vi "XYZStage-Z-axis safety interlock.vi"(7 "Interlock check type":T1, 8 "error in (no error)":errorcluster, 10 "Z move to":sgl, 11 "Z Current":sgl) -> (0 "error out":errorcluster, 3 "Z":sgl)   [LabVIEW 2020]
uses:
  Typedefs/Z intelock check type.ctl
  User Interface/Windows/Position control window/Globals/Pos ctrl window globals.vi
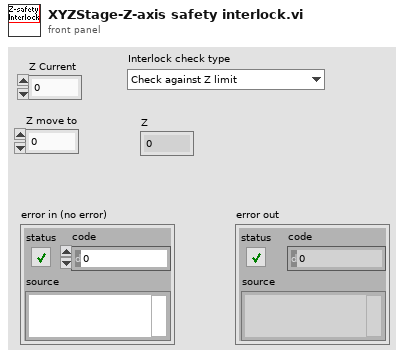
[diagram p1: front panel]
types:
  T1 = typedef "Z intelock check type.ctl" = enum16{"Check against Z limit", "Check againt current position"}
  T2 = typedef "Imaging Protocols enum.ctl" = enum16{"AOL Z-Stack", "Motor Z Stack", "Parameter Sweep", "Functional Acquisition", "Single Plane Acquisition", "Volume Acquisition", "Live Imaging", "Live Plane Imaging", "Live Volume Imaging"}
  T3 = cluster{"Caption-Right button":string, "Caption-Left button":string, "Message to display":string, "Delay before close":u32, "Window Colour":u32, "Cancel button disabled?":enum8{"Enabled", "Disabled", "Disabled and Grayed Out"}}
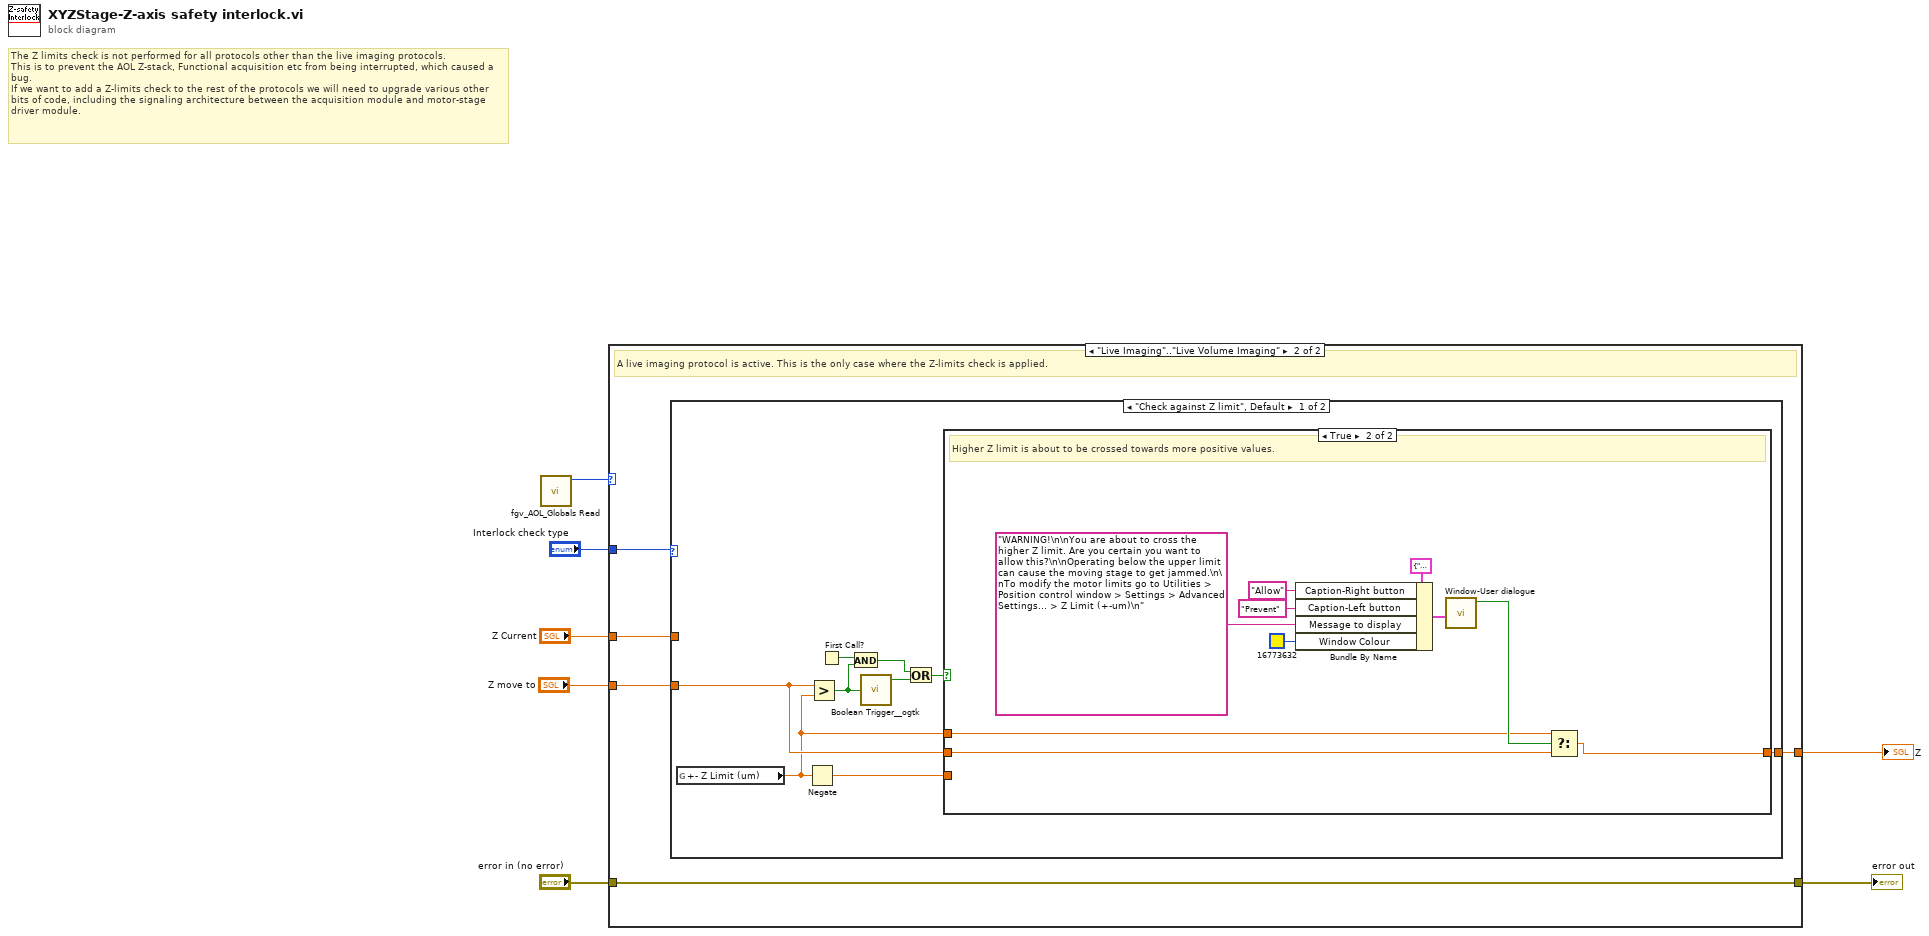
[diagram p0: block diagram]
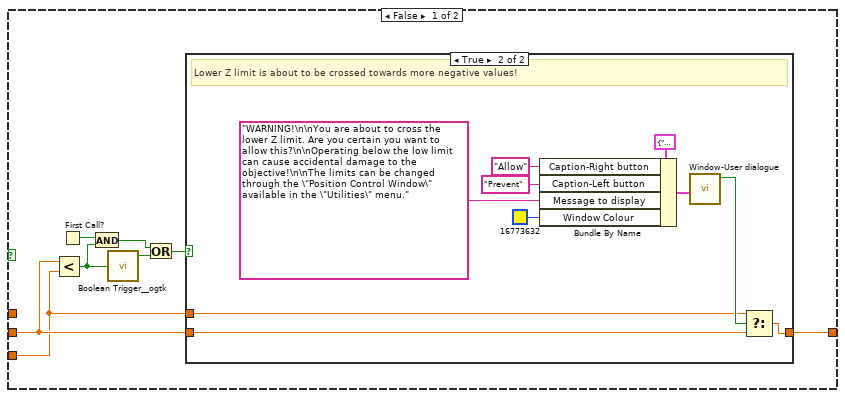
[diagram p3: hidden frame]
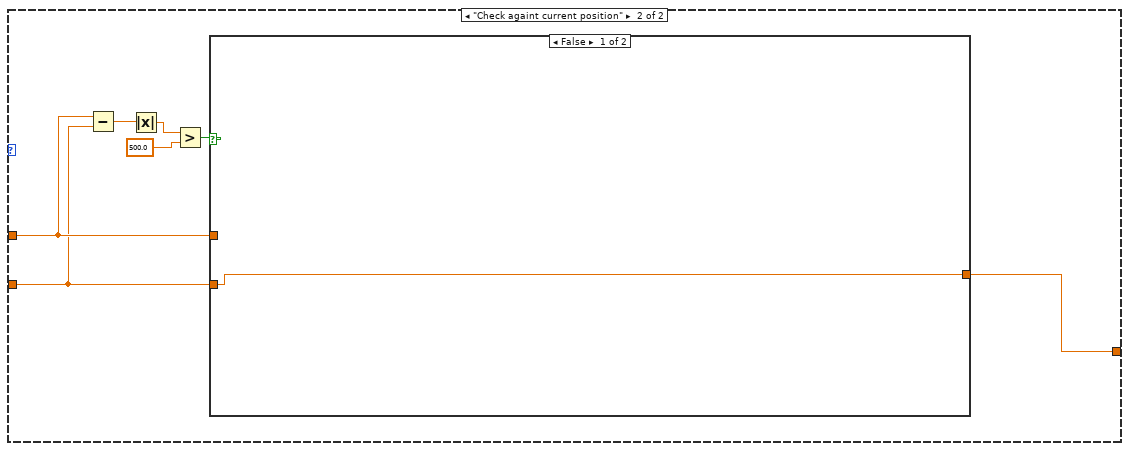
[diagram p5: hidden frame]
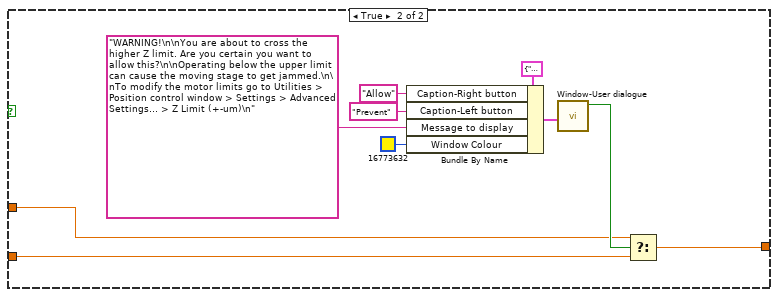
[diagram p6: hidden frame]
diagram:
  # "The Z limits check is not performed for all protocols other than the live imaging protocols.\nThis is to prevent the AOL Z-stack, Functional acquisition etc from being interrupted, which caused a bug.\nIf we want to add a Z-limits check to the rest of the protocols we will need to upgrade various other bits of code, including the signaling architecture between the acquisition module and motor-stage driver module."
  n1 = call "fgv_AOL_Globals Read.vi"() -> ("Imaging Protocol"=w5:T2)  [unwired: 9 in, 2 out]
  n2 = case shown="\"Live Imaging\"..\"Live Volume Imaging\"" w5 {
    tunnel: [w9 w14] -> w7
    tunnel: "Z move to" -> [w9 w13]
    tunnel: "Interlock check type" -> [_ w12]
    tunnel: "Z Current" -> [_ w11]
    tunnel: [w8 w10] -> w1
    tunnel: "error in (no error)" -> [w8 w10]
    frame Default {
      # "Do nothing. No Z-limits check for all protocols other than the live imaging protocols."
    }
    frame "Live Imaging".."Live Volume Imaging" {
      # "A live imaging protocol is active. This is the only case where the Z-limits check is applied."
      n3 = case shown="\"Check against Z limit\", Default" w12 {
        tunnel: [w23 w53] -> w14
        tunnel: w13 -> [w22 w54]
        tunnel: w11 -> [_ w55]
        frame "Check against Z limit", Default {
          n4 = global read "Pos ctrl window globals.vi" "+- Z Limit (um)"() -> (w21:sgl)
          n5 = Negate(x=w21) -> (-x=w20:sgl)
          n6 = Greater?(x=w22, y=w21) -> (0:w18:bool)
          n7 = First Call?() -> (First Call?: T/F=w19:bool)
          n8 = And(x=w19, y=w18) -> (x .and. y?=w16:bool)
          n9 = call <userlib>:"Boolean Trigger__ogtk.vi"("Boolean Input"=w18) -> ("Rising Edge"=w17:bool)  [unwired: 1 in, 1 out]
          n10 = Or(x=w16, y=w17) -> (x .or. y?=w15:bool)
          n11 = case shown="True" w15 {
            tunnel: w22 -> [w30 w52]
            tunnel: [w31 w51] -> w23
            tunnel: w21 -> [_ w49]
            tunnel: w20 -> [w29 _]
            frame False {
              n12 = Less?(x=w30, y=w29) -> (x < y?=w28:bool)
              n13 = First Call?() -> (First Call?: T/F=w27:bool)
              n14 = And(x=w27, y=w28) -> (x .and. y?=w24:bool)
              n15 = call <userlib>:"Boolean Trigger__ogtk.vi"("Boolean Input"=w28) -> ("Rising Edge"=w26:bool)  [unwired: 1 in, 1 out]
              n16 = Or(x=w24, y=w26) -> (x .or. y?=w25:bool)
              n17 = case shown="True" w25 {
                tunnel: w30 -> [w32 w42]
                tunnel: [w32 w41] -> w31
                tunnel: w29 -> [_ w39]
                frame False {
                }
                frame True {
                  # "Lower Z limit is about to be crossed towards more negative values!"
                  n18 = Bundle By Name(cluster=T3 {"Caption-Right button"="", "Caption-Left button"="", "Message to display"="", "Delay before close"=0, "Window Colour"=16448250, "Cancel button disabled?"=enum."Enabled"} ("Input cluster"), "Caption-Right button"="Allow", "Caption-Left button"="Prevent", "Message to display"="WARNING!\n\nYou are about to cross the lower Z limit. Are you certain you want to allow this?\n\nOperating below the low limit can cause accidental damage to the objective!\n\nThe limits can be changed through the \"Position Control Window\" available in the \"Utilities\" menu." ("Message string"), "Window Colour"=u32 16773632) -> (w34:T3)
                  n19 = call "Window-User dialogue.vi"("Input cluster"=w34) -> ("Left Button (Cancel)"=w40:bool)  [unwired: 10 in]
                  n20 = Select(t=w39, s=w40, f=w42) -> (s? t:f=w41:sgl)
                }
              }
            }
            frame True {
              # "Higher Z limit is about to be crossed towards more positive values."
              n21 = Bundle By Name(cluster=T3 {"Caption-Right button"="", "Caption-Left button"="", "Message to display"="", "Delay before close"=0, "Window Colour"=16448250, "Cancel button disabled?"=enum."Enabled"} ("Input cluster"), "Caption-Right button"="Allow", "Caption-Left button"="Prevent", "Message to display"="WARNING!\n\nYou are about to cross the higher Z limit. Are you certain you want to allow this?\n\nOperating below the upper limit can cause the moving stage to get jammed.\n\nTo modify the motor limits go to Utilities > Position control window > Settings > Advanced Settings… > Z Limit (+-um)\n" ("Message string"), "Window Colour"=u32 16773632) -> (w44:T3)
              n22 = call "Window-User dialogue.vi"("Input cluster"=w44) -> ("Left Button (Cancel)"=w50:bool)  [unwired: 10 in]
              n23 = Select(t=w49, s=w50, f=w52) -> (s? t:f=w51:sgl)
            }
          }
        }
        frame "Check againt current position" {
          n24 = Subtract(x=w55, y=w54) -> (x-y=w59:sgl)
          n25 = Absolute Value(x=w59) -> (abs(x)=w58:sgl)
          n26 = Greater?(x=w58, y=sgl 500.0) -> (0:w56:bool)
          n27 = case shown="False" w56 {
            tunnel: w55 -> [_ w63]
            tunnel: w54 -> [w60 w62]
            tunnel: [w60 w61] -> w53
            frame False {
            }
            frame True {
              n28 = Bundle By Name(cluster=T3 {"Caption-Right button"="", "Caption-Left button"="", "Message to display"="", "Delay before close"=0, "Window Colour"=16448250, "Cancel button disabled?"=enum."Enabled"} ("Input cluster"), "Caption-Right button"="Allow", "Caption-Left button"="Prevent", "Message to display"="WARNING!\n\nYou are about to cross the higher Z limit. Are you certain you want to allow this?\n\nOperating below the upper limit can cause the moving stage to get jammed.\n\nTo modify the motor limits go to Utilities > Position control window > Settings > Advanced Settings… > Z Limit (+-um)\n" ("Message string"), "Window Colour"=u32 16773632) -> (w66:T3)
              n29 = call "Window-User dialogue.vi"("Input cluster"=w66) -> ("Left Button (Cancel)"=w64:bool)  [unwired: 10 in]
              n30 = Select(t=w63, s=w64, f=w62) -> (s? t:f=w61:sgl)
            }
          }
        }
      }
    }
  }
  "Z" <- w7
  "error out" <- w1
